vi "Serial port setup.vi"(11 "Serial Configuration":T1={"Baud Rate"=9600, "Parity"=2, "Data Bits"=7, "VISA resource name"=""} {"Data Bits" items=["7"=7, "8"=8]; "Parity" items=["None", "Odd", "Even"]; "Baud Rate" items=["300"=300, "600"=600, "1200"=1200, "2400"=2400, "4800"=4800, "9600"=9600, "19200"=19200]}) -> (0 "error out":errorcluster, 3 "VISA resource name out":refnum<visa-resource-name>)   [LabVIEW 2018]
uses:
  Serial configuration cluster control.ctl
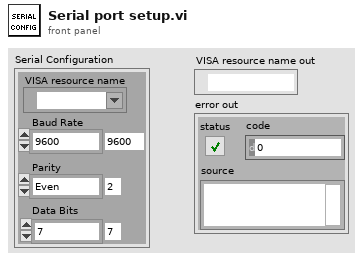
[diagram p1: front panel]
types:
  T1 = typedef "Serial configuration cluster control.ctl" = cluster{"Baud Rate":u32, "Parity":u16, "Data Bits":u16, "VISA resource name":refnum<visa-resource-name>}
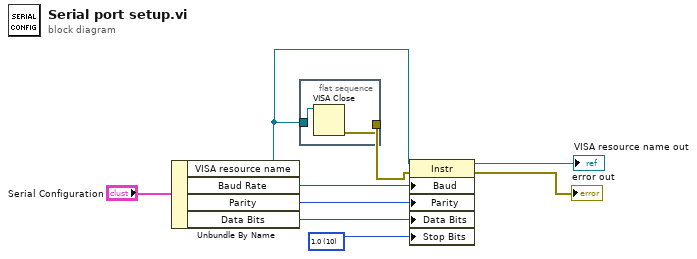
[diagram p0: block diagram]
diagram:
  w5 = u16 10 items=["1.0"=10, "1.5"=15, "2.0"=20] ("Serial Settings:Stop Bits")
  n1 = Unbundle By Name("Serial Configuration") -> ("VISA resource name"=w2:refnum<visa-resource-name>, "Baud Rate"=w8:u32, "Parity"=w7:u16, "Data Bits"=w6:u16)
  n2 = flat-sequence {
    tunnel: w2 -> [w11]
    tunnel: [w10] -> w1
    frame #0 {
      n3 = VISA Close(VISA resource name=w11) -> (error out=w10:errorcluster)  [unwired: 1 in]
    }
  }
  n4 = property class="Instr"(reference=w2, error in=w1, "Baud"=w8, "Parity"=w7, "Data Bits"=w6, "Stop Bits"=w5) -> (reference out=→"VISA resource name out":refnum<visa-resource-name>, error out=→"error out":errorcluster)
